vi "WFGenerate.vi"(8 "error in (no error)":errorcluster, 11 "Stimulus Type":u16(ring) items=["Off", "DC", "Noise", "PT", "FM"]) -> (0 "error out":errorcluster, 3 "Waveform Out":waveform(dbl))   [LabVIEW 2009]
panel:
  in  "Repetitions":T1 {"Interval (s)" min=0.0; "Delay (s)" min=0.0}
  in  "Waveform Parameters":T2
  in  "Waveform Properties":T3 {"Ramp (s)" min=0.0; "Fs (Hz)" min=0.0}
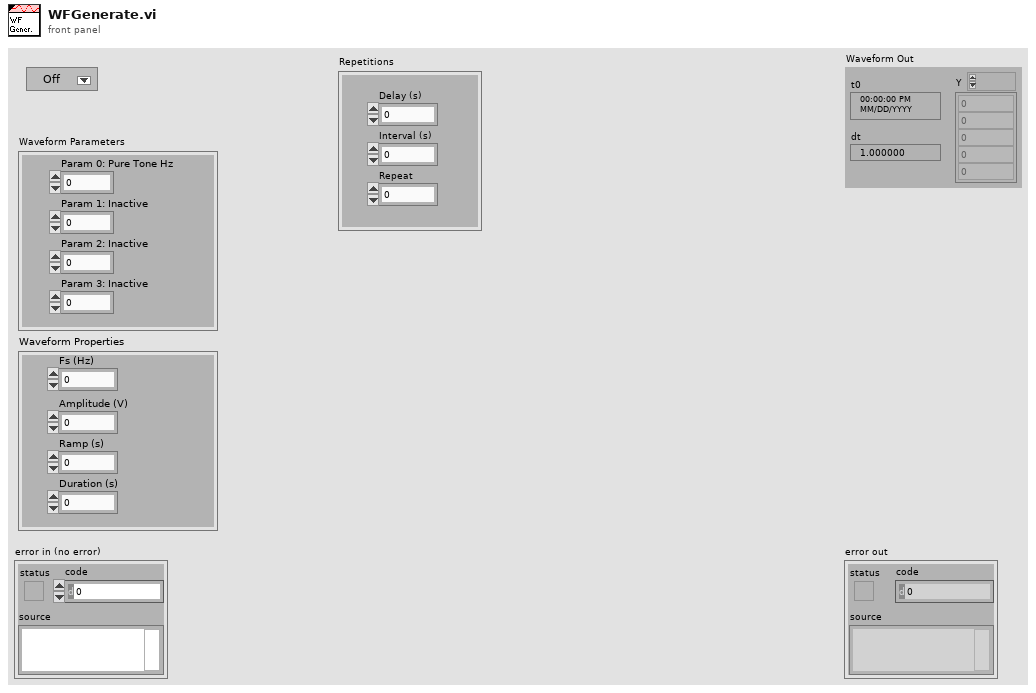
[diagram p1: front panel]
types:
  T1 = cluster{"Delay (s)":dbl, "Interval (s)":dbl, "Repeat":i32}
  T2 = cluster{"Param 0: Pure Tone Hz":dbl, "Param 1: Inactive":dbl, "Param 2: Inactive":dbl, "Param 3: Inactive":dbl}
  T3 = cluster{"Fs (Hz)":dbl, "Amplitude (V)":dbl, "Ramp (s)":dbl, "Duration (s)":dbl}
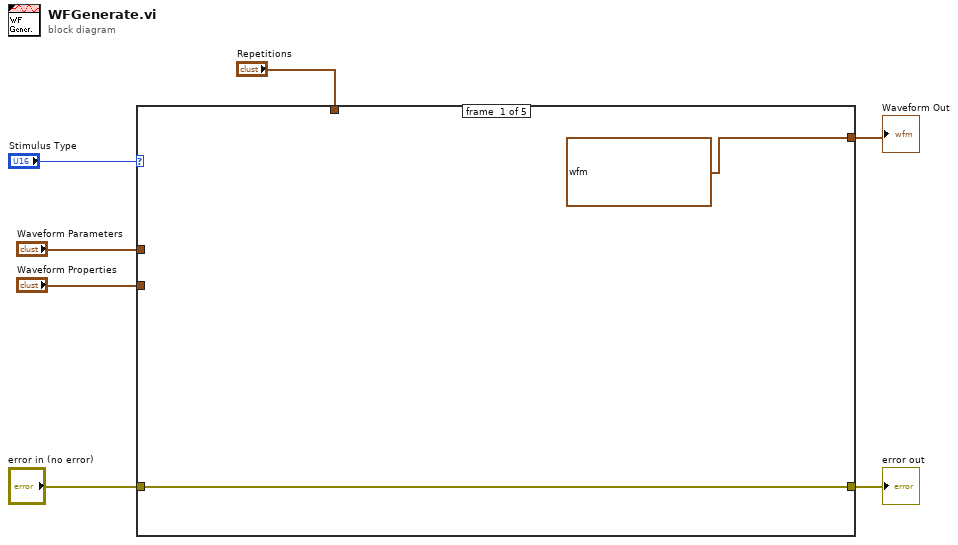
[diagram p0: block diagram]
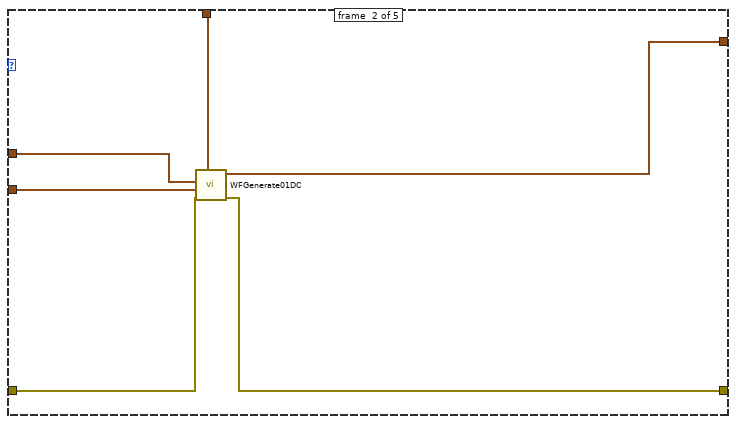
[diagram p2: hidden frame]
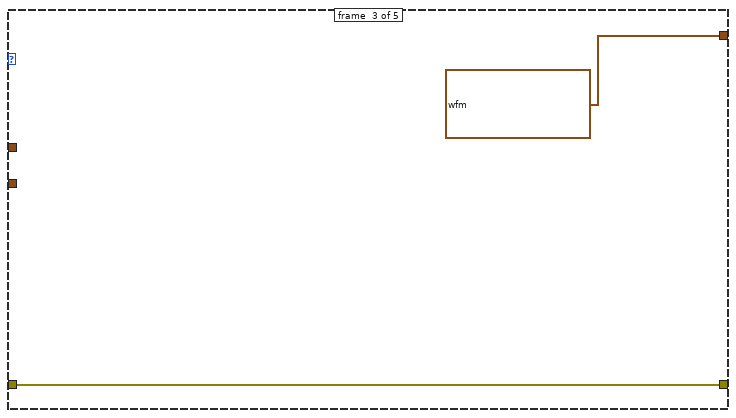
[diagram p3: hidden frame]
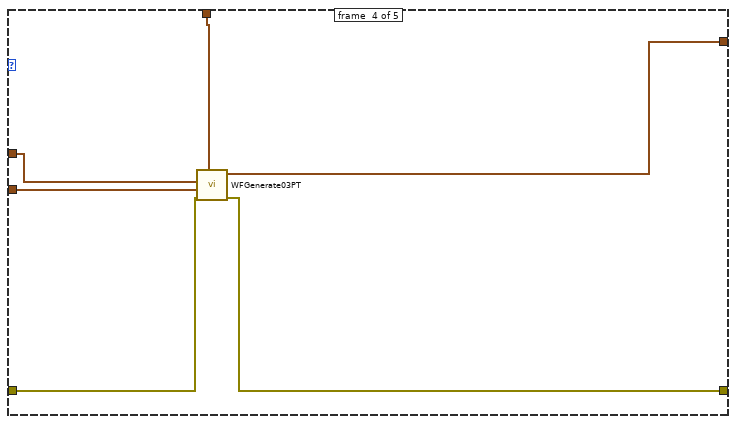
[diagram p4: hidden frame]
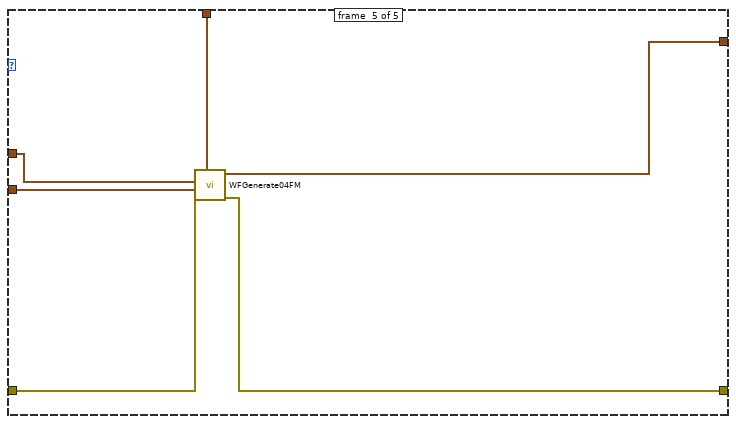
[diagram p5: hidden frame]
diagram:
  n1 = case shown="4" "Stimulus Type" {
    tunnel: "error in (no error)" -> [w8 w15 w17 w23 w29]
    tunnel: [w8 w14 w17 w22 w28] -> w5
    tunnel: [waveform(dbl) ? ("Waveform") w13 waveform(dbl) ? ("Waveform") w21 w27] -> w4
    tunnel: "Repetitions" -> [_ w12 _ w20 w26]
    tunnel: "Waveform Parameters" -> [_ w11 _ w18 w24]
    tunnel: "Waveform Properties" -> [_ w10 _ w19 w25]
    frame #0 {
    }
    frame #1 {
      n2 = call "WFGenerate01DC.vi"("Repetitions"=w12, "error in (no error)"=w15, "Waveform Properties"=w10, "Waveform Parameters"=w11) -> ("error out"=w14:errorcluster, "Waveform Out"=w13:waveform(dbl))  [unwired: 6 in]
    }
    frame #2 {
    }
    frame #3 {
      n3 = call "WFGenerate03PT.vi"("Repetitions"=w20, "error in (no error)"=w23, "Waveform Properties"=w19, "Waveform Parameters"=w18) -> ("error out"=w22:errorcluster, "Waveform Out"=w21:waveform(dbl))  [unwired: 6 in]
    }
    frame #4 {
      n4 = call "WFGenerate04FM.vi"("Repetitions"=w26, "error in (no error)"=w29, "Waveform Properties"=w25, "Waveform Parameters"=w24) -> ("error out"=w28:errorcluster, "Waveform Out"=w27:waveform(dbl))  [unwired: 6 in]
    }
  }
  "Waveform Out" <- w4
  "error out" <- w5
